vi "TCP.IP Server for Ripple Detection - exp.vi"() -> ()   [LabVIEW 2021]
doc: "Demonstrates how to set up a basic TCP connection, send data to the specified port once a connection has been established, and terminate the connection once the data has been sent. This VI is designed to stop if the TCP connection is terminated. The data sent in this example is an array of random numbers."
panel:
  out "Waveform Graph 10":dbl[](graph)
  in  "loop 1":i32
  in  "Client Closed":string="The client VI closed the connection."
  in  "Stop":bool
  # "Overview: Demonstrates the use of the TCP functions to initialize a TCP server that can send data to a client VI.\nInstructions:\n1. Run the VI.\n2. Open Simple TCP - Client.vi and follow the instructions on its front panel. Note that if you wait longer than 30 seconds to do this after running this VI, it will time out.\n3. Click Stop to stop the VI. Note that if you stop the client VI, this VI will stop automatically."
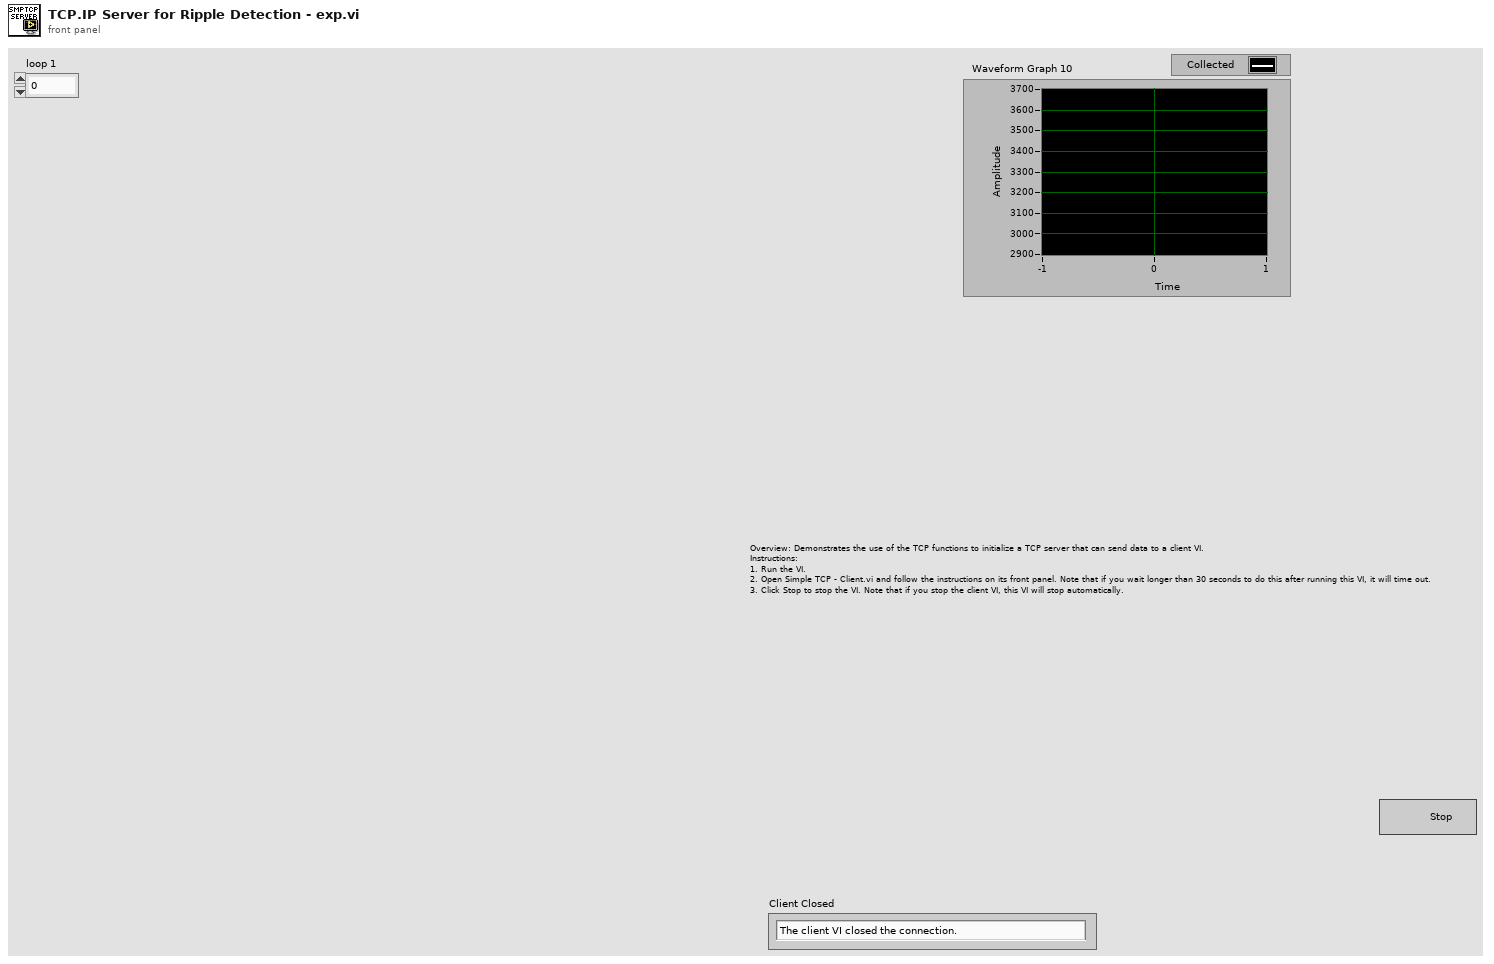
[diagram p1: front panel]
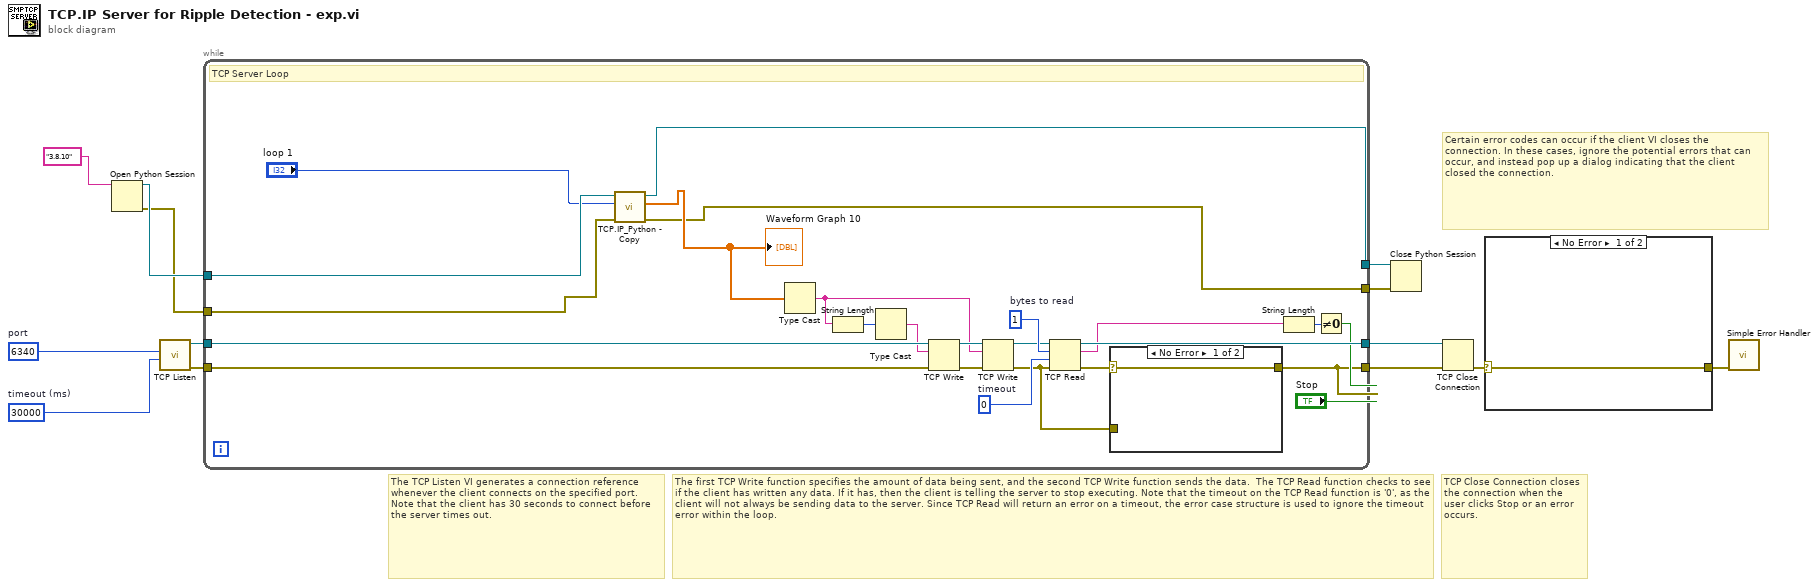
[diagram p0: block diagram]
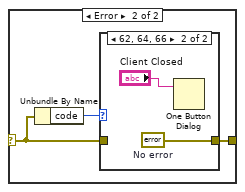
[diagram p2: hidden frame]
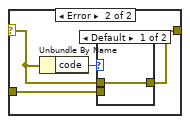
[diagram p4: hidden frame]
diagram:
  w6 = u16 6340  # port
  w7 = 30000  # timeout (ms)
  # "TCP Close Connection closes the connection when the user clicks Stop or an error occurs."
  # "The TCP Listen VI generates a connection reference whenever the client connects on the specified port. Note that the client has 30 seconds to connect before the server times out."
  # "Certain error codes can occur if the client VI closes the connection. In these cases, ignore the potential errors that can occur, and instead pop up a dialog indicating that the client closed the connection."
  # "The first TCP Write function specifies the amount of data being sent, and the second TCP Write function sends the data.  The TCP Read function checks to see if the client has written any data. If it has, then the client is telling the server to stop executing. Note that the timeout on the TCP Read function is '0', as the client will not always be sending data to the server. Since TCP Read will return an error on a timeout, the error case structure is used to ignore the timeout error within the loop."
  n1 = Open Python Session(python version="3.8.10" ("Python version")) -> (session out=w4:refnum<k35>, error out=w3:errorcluster)  [unwired: 2 in]
  n2 = call <vilib>:"TCP Listen.vi"("timeout ms (wait forever: -1)"=w7, "port"=w6) -> ("error out"=w8:errorcluster, "connection ID"=w9:refnum<k5>)  [unwired: 5 in, 3 out]
  n3 = while {
    tunnel: [w21] -> w12
    tunnel: [w27] -> w13
    tunnel: w9 -> [w38]
    tunnel: w8 -> [w31]
    tunnel: w4 -> [w15]
    tunnel: w3 -> [w16]
    tunnel: [w19] -> w2
    tunnel: [w17] -> w1
    stop <- w32 stop-if-true
    w26 = 0  # timeout
    w29 = 1  # bytes to read
    # "TCP Server Loop"
    n4 = call "TCP.IP_Python - Copy.vi"("error in (no error)"=w16, "loop 1"="loop 1", "Refnum in"=w15) -> ("error out"=w17:errorcluster, "Array"=w18:dbl[], "Refnum out"=w19:refnum<k35>)  [unwired: 6 in]
    "Waveform Graph 10" <- w18
    n5 = Type Cast(x=w18) -> (*(type *) &x=w33:string)  [unwired: 1 out]
    n6 = String Length(string=w33) -> (length=w35:i32)
    n7 = Type Cast(x=w35) -> (*(type *) &x=w34:string)  [unwired: 1 out]
    n8 = TCP Write(connection ID=w38, data in=w34, error in (no error)=w31) -> (connection ID out=w37:refnum<k5>, error out=w36:errorcluster)  [unwired: 2 out]
    n9 = TCP Write(connection ID=w37, data in=w33, error in (no error)=w36) -> (connection ID out=w28:refnum<k5>, error out=w20:errorcluster)  [unwired: 2 out]
    n10 = TCP Read(connection ID=w28, bytes to read=w29, error in (no error)=w20, 9:w26) -> (connection ID out=w27:refnum<k5>, data out=w24:string, error out=w22:errorcluster)  [unwired: 1 out]
    n11 = case shown="No Error" w22 {
      selector: w22 -> [w39 w42]
      tunnel: [w39 w40] -> w21
      tunnel: w20 -> [_ w41]
      frame No Error {
      }
      frame Error {
        n12 = Unbundle By Name(w42) -> ("code"=w43:i32)
        n13 = case shown="Default" w43 {
          tunnel: w42 -> [w44 _]
          tunnel: w41 -> [_ w45]
          tunnel: [w44 w45] -> w40
          frame Default {
          }
          frame 56 {
          }
        }
      }
    }
    n14 = String Length(string=w24) -> (length=w25:i32)
    n15 = Not Equal To 0?(x=w25) -> (x != 0?=w23:bool)
    n16 = Compound Arithmetic op=OR(w23, w21, "Stop") -> (w32:bool)
  }
  n17 = Close Python Session(session in=w2, error in=w1) -> ()  [unwired: 1 out]
  n18 = TCP Close Connection(connection ID=w13, error in (no error)=w12) -> (error out=w11:errorcluster)  [unwired: 2 out]
  n19 = case shown="No Error" w11 {
    selector: w11 -> [w46 w48]
    tunnel: [w46 w47] -> w10
    frame No Error {
    }
    frame Error {
      n20 = Unbundle By Name(w48) -> ("code"=w49:i32)
      n21 = case shown="62, 64, 66" w49 {
        tunnel: w48 -> [w50 _]
        tunnel: [w50 w52] -> w47
        frame Default {
        }
        frame 62, 64, 66 {
          w52 = errorcluster {"status"=FALSE, "code"=0, "source"=""}  # No error
          n22 = One Button Dialog(message="Client Closed") -> ()  [unwired: 1 in, 1 out]
        }
      }
    }
  }
  n23 = call <vilib>:"Simple Error Handler.vi"("error in (no error)"=w10) -> ()  [unwired: 1 in, 8 out]
